vi "kafkaStream_Write.vi"(0 "Kafka Producer Handle":string, 1 "File Name":string="untitled", 2 "Kafka Partition":u32, 5 "Group Name":string, 7 "Channel Names":string[](array[string]), 9 "Waveforms":waveform(dbl)[](array[waveform]), 11 "error in (no error)":errorcluster, 12 "Property Names":string[][](array[string]), 13 "Debug":bool, 14 "Property Values":variant[][](array[variant])) -> (3 "File Name Out":string="untitled", 4 "Kafka Producer Handle Out":string, 6 "Group Name Out":string, 8 "Channel Names Out":string[](array[string]), 15 "error out":errorcluster)   [LabVIEW 2019]
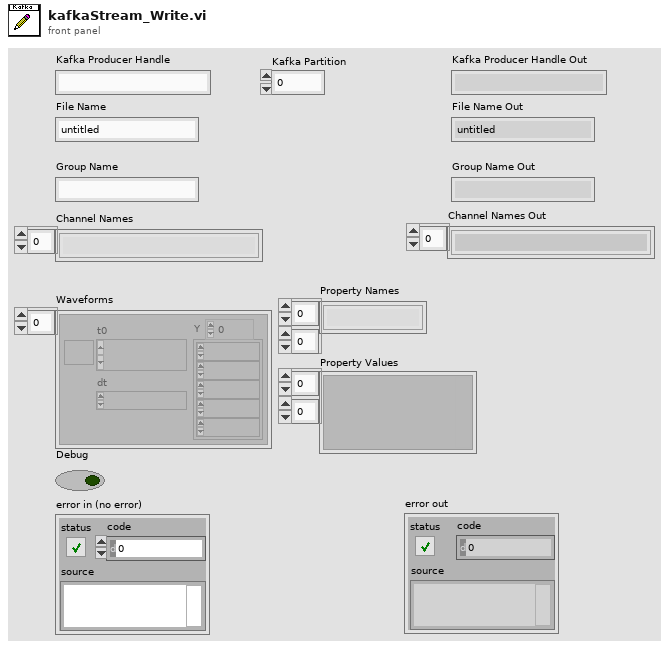
[diagram p1: front panel]
types:
  T1 = typedef "KafkaConsumerEvent.ctl" = cluster{"Payload":string, "Key":string, "MsgLen":u64, "Offset":i64, "Time Stamp":i64, "TS Name":string}
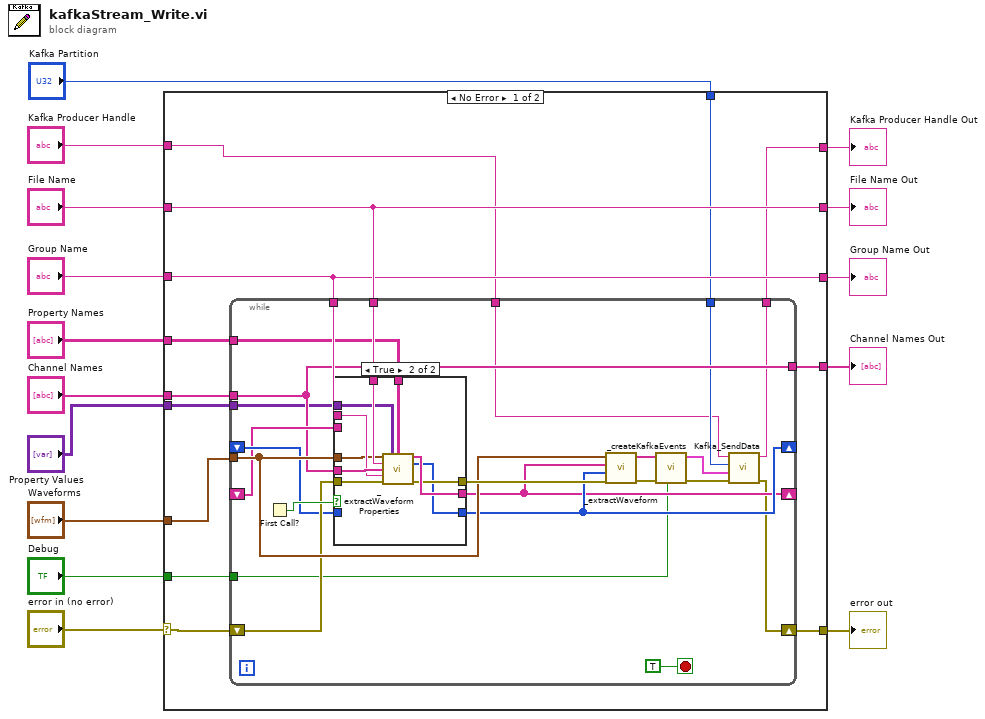
[diagram p0: block diagram]
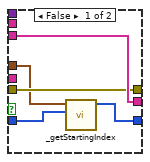
[diagram p2: hidden frame]
diagram:
  n1 = case shown="No Error" "error in (no error)" {
    selector: "error in (no error)" -> [w28 w71]
    tunnel: "Group Name" -> [w23 w69]
    tunnel: "Channel Names" -> [w25 w70]
    tunnel: "Waveforms" -> [w26 _]
    tunnel: [w27 w71] -> w11
    tunnel: "File Name" -> [w24 w68]
    tunnel: [w22 w70] -> w9
    tunnel: [w23 w69] -> w8
    tunnel: [w24 w68] -> w7
    tunnel: "Kafka Partition" -> [w21 _]
    tunnel: "Kafka Producer Handle" -> [w20 w67]
    tunnel: [w19 w67] -> w4
    tunnel: "Debug" -> [w18 _]
    tunnel: "Property Values" -> [w17 _]
    tunnel: "Property Names" -> [w16 _]
    frame No Error {
      n2 = while {
        shift-right: [w35] -> w27
        shift-left: w28 -> [w47]
        tunnel: w26 -> [w48]
        tunnel: w25 -> [w40]
        tunnel: w23 -> [w46]
        shift-right: [w45] -> _
        shift-left: _ -> [w44]
        shift-right: [w43] -> _
        shift-left: _ -> [w42]
        tunnel: w24 -> [w41]
        tunnel: [w40] -> w22
        tunnel: w21 -> [w37]
        tunnel: w20 -> [w36]
        tunnel: [w32] -> w19
        tunnel: w18 -> [w31]
        tunnel: w17 -> [w30]
        tunnel: w16 -> [w29]
        stop <- TRUE stop-if-true
        n3 = First Call?() -> (First Call?: T/F=w50:bool)
        n4 = case shown="True" w50 {
          tunnel: w48 -> [w54 w60]
          tunnel: w47 -> [w55 w66]
          tunnel: w40 -> [_ w65]
          tunnel: w46 -> [_ w63]
          tunnel: w41 -> [_ w64]
          tunnel: [w56 w62] -> w43
          tunnel: w42 -> [w56 _]
          tunnel: [w55 w61] -> w51
          tunnel: [w53 w59] -> w45
          tunnel: w44 -> [w52 _]
          tunnel: w30 -> [_ w58]
          tunnel: w29 -> [_ w57]
          frame False {
            n5 = call "_getStartingIndex.vi"("Starting Index In"=w52, "Waveforms"=w54) -> ("Starting Index"=w53:u32[])  [unwired: 9 in]
          }
          frame True {
            n6 = call "_extractWaveformProperties.vi"("Waveforms"=w60, "Property Values"=w58, "Property Names"=w57, "File Name"=w64, "Channel Names"=w65, "Group Name"=w63, "error in (no error)"=w66) -> ("Event Object"=w62:string[], "Starting Index Increment"=w59:u32[], "error out"=w61:errorcluster)  [unwired: 6 in]
          }
        }
        n7 = call "_extractWaveform.vi"("Waveforms"=w48, "Event Object In"=w43, "Starting Index"=w45, "error in (no error)"=w51) -> ("Event Object Out"=w33:string[], "error out"=w34:errorcluster)  [unwired: 5 in]
        n8 = call "_createKafkaEvents.vi"("Payload"=w33, "error in (no error)"=w34, "Debug"=w31) -> ("Kafka Events"=w39:T1[], "error out"=w38:errorcluster)  [unwired: 6 in]
        n9 = call "Kafka_SendData.vi"("error in (no error)"=w38, "Events"=w39, "Partition"=w37, "Producer Handle"=w36) -> ("error out"=w35:errorcluster, "Producer Handle"=w32:string)  [unwired: 6 in]
      }
    }
    frame Error {
    }
  }
  "error out" <- w11
  "Channel Names Out" <- w9
  "Group Name Out" <- w8
  "File Name Out" <- w7
  "Kafka Producer Handle Out" <- w4
